vi "Fattore Ko correz temp.vi"(7 "Rame?":bool=TRUE, 10 "T avvolg a fine prova (°C)":dbl, 11 "T fluido ingresso (°C)":dbl) -> (2 "Ko":dbl)   [LabVIEW 2019]
panel:
  # "fattore di correzione Kq della temperatura per gli avvolgimenti"
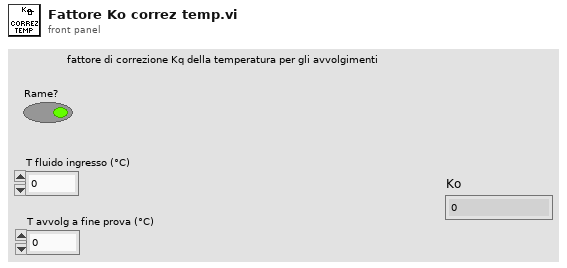
[diagram p1: front panel]
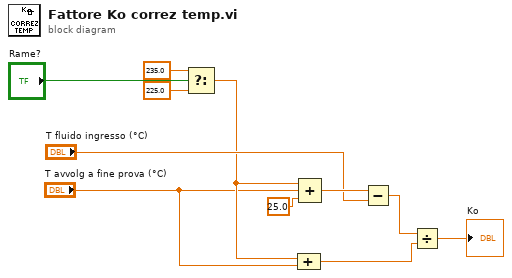
[diagram p0: block diagram]
diagram:
  n1 = Select(t=235.0, s="Rame?", f=225.0) -> (s? t:f=w4:dbl)
  n2 = Compound Arithmetic op=ADD(w4, "T avvolg a fine prova (°C)") -> (w2:dbl)
  n3 = Compound Arithmetic op=ADD(w4, "T avvolg a fine prova (°C)", 25.0 ("value")) -> (w7:dbl)
  n4 = Subtract(x=w7, y="T fluido ingresso (°C)") -> (x-y=w5:dbl)
  n5 = Divide(x=w5, y=w2) -> (x/y=→"Ko":dbl)
